vi "StringToDataWaveform.vi"() -> ()   [LabVIEW 2021]
uses:
  <vilib>/measure/NI_MABase.lvlib
panel:
  out "Waveform Chart 2":dbl[](graph)
  in  "Freq":dbl(knob) scale=0.0..100.0
  out "Waveform Chart":i16[](graph)
  out "Array":i16[](array[numeric])
  out "ASCII Number of String":u8[](array[numeric])
  in  "String":string
  # "Convert Name into signal\nModulize the Data"
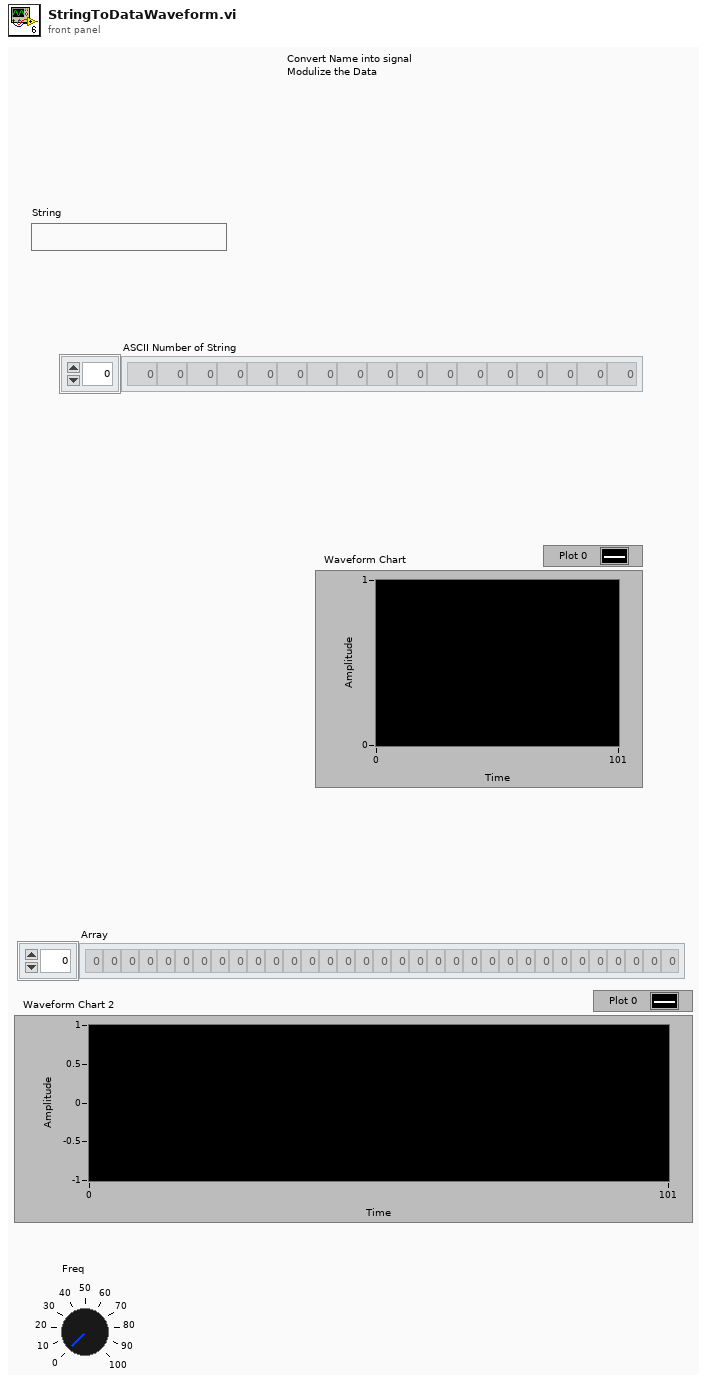
[diagram p1: front panel]
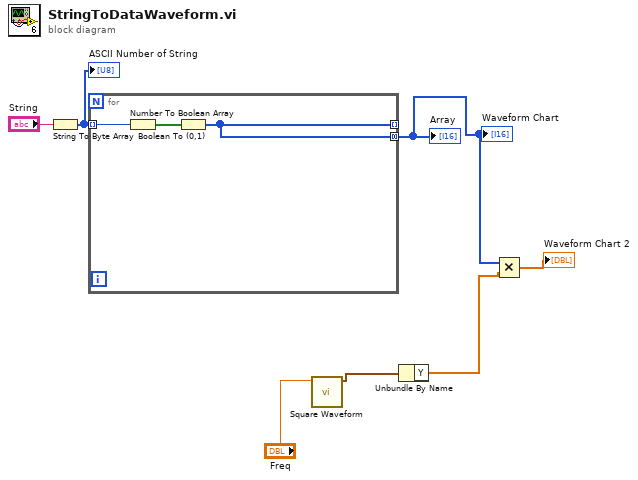
[diagram p0: block diagram]
diagram:
  n1 = String To Byte Array(string="String") -> (unsigned byte array=w6:u8[])
  "ASCII Number of String" <- w6
  n2 = for {
    tunnel: w6 -> [w10] mode=indexing
    tunnel: [w8] -> _ mode=indexing
    tunnel: [w8] -> w5 mode=concatenating
    n3 = Number To Boolean Array(number=w10) -> (Boolean array=w9:bool[])
    n4 = Boolean To (0,1)(Boolean=w9) -> (0, 1=w8:i16[])
  }
  "Array" <- w5
  "Waveform Chart" <- w5
  n5 = call <vilib>:"Square Waveform.vi"("frequency"="Freq") -> ("signal out"=w3:waveform(dbl))  [unwired: 9 in, 1 out]
  n6 = Unbundle By Name(w3) -> ("Y"=w2:dbl[])
  n7 = Multiply(x=w5, y=w2) -> (x*y=→"Waveform Chart 2":dbl[])
